vi "SRXConfigLimitSwitchSingle.vi"(0 "PhoenixMotorControlDevRefIn":T1={"DeviceStatus"={"status"=FALSE, "code"=0, "source"=""}, "Type"=enum."PWM", "PWM"={"PWM Channel"=enum."PWM 1", "DeadBand"={"Name"="", "maxPositivePwm"=0, "minPositivePwm"=0, "centerPwm"=0, "maxNegativePwm"=0, "minNegativePwm"=0, "angularRange"=0}}, "CAN"={"Device Number"=0, "SetOutput VI Ref"=variant(enum8{"Percent VBus", "Current", "Speed", "Position", "Voltage"} enum."Percent VBus"), "GetOutput VI Ref"=variant(refnum<k1> refnum), "Enable VI Ref"=variant(dbl 12.0), "Disable VI Ref"=variant(enum8{"Percent VBus", "Speed", "Position", "Slave", "Unchanged / Invalid", "Voltage Compensation", "Current", "Motion Profile"} enum."Percent VBus"), "Data"=variant}, "Invert"=FALSE, "DIO PWM"={"PWM \"Enable\" Channel"=enum."Invalid", "DIOChannel"=enum."Invalid", "PWM Rate"=0.0}}, 5 "MotorConfig":T6={"CAN Address"=0, "Invert"=FALSE, "InvertSensor"=FALSE, "Unit Conversion Factor"=0.0, "Brake Mode"=enum."Override to Brake", "Reverse Limt Switch Mode"=enum."Disabled", "Forward Limt Swith Mode"=enum."Disabled", "PWM Channel"=enum."Invalid", "Motor Controller Type"=enum."Talon SRX"}, 11 "error in (no error)":errorcluster) -> (4 "PhoenixMotorControlDevRefOut":T1={"DeviceStatus"={"status"=FALSE, "code"=0, "source"=""}, "Type"=enum."PWM", "PWM"={"PWM Channel"=enum."PWM 1", "DeadBand"={"Name"="", "maxPositivePwm"=0, "minPositivePwm"=0, "centerPwm"=0, "maxNegativePwm"=0, "minNegativePwm"=0, "angularRange"=0}}, "CAN"={"Device Number"=0, "SetOutput VI Ref"=variant(enum8{"Percent VBus", "Current", "Speed", "Position", "Voltage"} enum."Percent VBus"), "GetOutput VI Ref"=variant(refnum<k1> refnum), "Enable VI Ref"=variant(dbl 12.0), "Disable VI Ref"=variant(enum8{"Percent VBus", "Speed", "Position", "Slave", "Unchanged / Invalid", "Voltage Compensation", "Current", "Motion Profile"} enum."Percent VBus"), "Data"=variant}, "Invert"=FALSE, "DIO PWM"={"PWM \"Enable\" Channel"=enum."Invalid", "DIOChannel"=enum."Invalid", "PWM Rate"=0.0}}, 15 "error out":errorcluster)   [LabVIEW 2017]
uses:
  TypeDefs/ConfigComponents/Config_Motor.ctl
  <vilib>/Rock Robotics/WPI/ThirdParty/Phoenix-LabVIEW/Motor Controller/Controls/CTRE_Phoenix_MotorControl_NeutralMode.ctl
  <vilib>/Rock Robotics/WPI/ThirdParty/Phoenix-LabVIEW/Motor Controller/Controls/CTRE_Phoenix_MotorControl_LimitSwitchNormal.ctl
  <vilib>/Rock Robotics/SystemInterfaces/DIO/FPGA_DIOPWMChannel.ctl
  TypeDefs/ConfigComponents/Config_MotorCtrlType.ctl
  <vilib>/Rock Robotics/WPI/MotorControl/WPI_MotorControlDeviceRef.ctl
  <vilib>/Rock Robotics/WPI/MotorControl/WPI_MotorControlType.ctl
  <vilib>/Rock Robotics/WPI/PWM/WPI_PWMDeadband.ctl
  <vilib>/Rock Robotics/SystemInterfaces/DIO/FPGA_DIOChannel.ctl
  <vilib>/Rock Robotics/WPI/ThirdParty/Phoenix-LabVIEW/Motor Controller/Controls/CTRE_Phoenix_MotorControl_LimitSwitchSource_Local.ctl
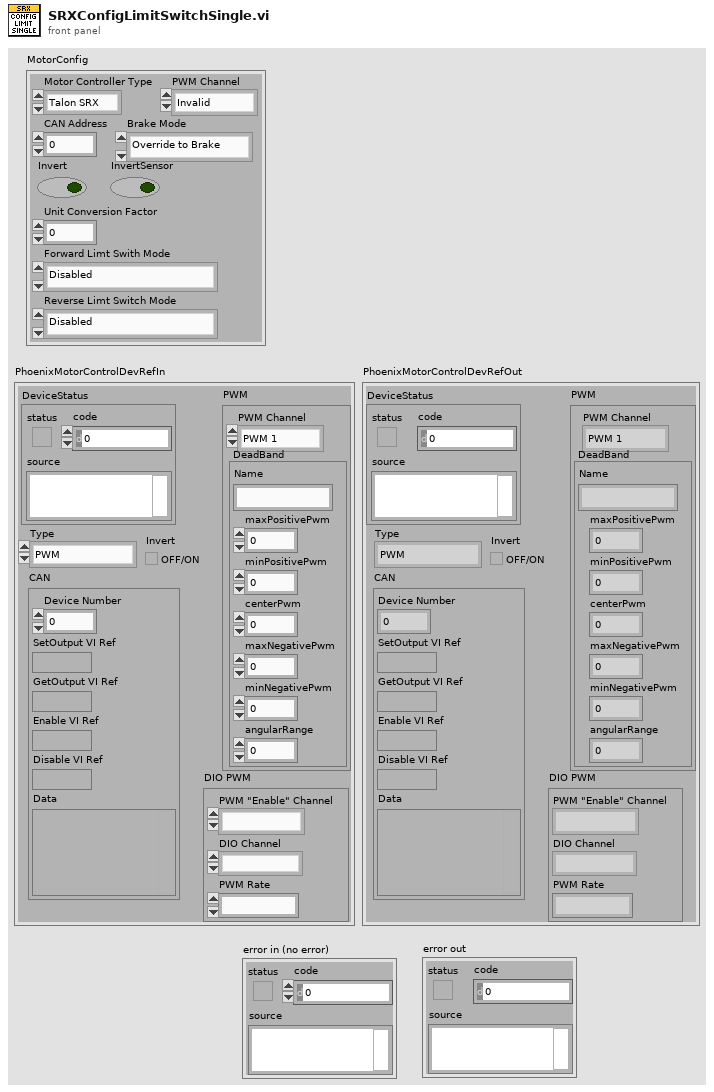
[diagram p1: front panel]
types:
  T1 = typedef "WPI_MotorControlDeviceRef.ctl" = cluster{"DeviceStatus":errorcluster, "Type":T2, "PWM":cluster{"PWM Channel":T3, "DeadBand":T4}, "CAN":cluster{"Device Number":u8, "SetOutput VI Ref":variant, "GetOutput VI Ref":variant, "Enable VI Ref":variant, "Disable VI Ref":variant, "Data":variant}, "Invert":bool, "DIO PWM":cluster{"PWM \"Enable\" Channel":T3, "DIOChannel":T5, "PWM Rate":dbl}}
  T2 = typedef "WPI_MotorControlType.ctl" = enum16{"PWM", "CAN", "DIO PWM"}
  T3 = typedef "FPGA_DIOPWMChannel.ctl" = enum8{"PWM 0", "PWM 1", "PWM 2", "PWM 3", "PWM 4", "PWM 5", "PWM 6", "PWM 7", "PWM 8", "PWM 9", "PWM MXP 0", "PWM MXP 1", "PWM MXP 2", "PWM MXP 3", "PWM MXP 4", "PWM MXP 5", "PWM MXP 6", "PWM MXP 7", "PWM MXP 8", "PWM MXP 9", "Invalid"}
  T4 = typedef "WPI_PWMDeadband.ctl" = cluster{"Name":string, "maxPositivePwm":i32, "minPositivePwm":i32, "centerPwm":i32, "maxNegativePwm":i32, "minNegativePwm":i32, "angularRange":u16}
  T5 = typedef "FPGA_DIOChannel.ctl" = enum8{"DIO 0", "DIO 1", "DIO 2", "DIO 3", "DIO 4", "DIO 5", "DIO 6", "DIO 7", "DIO 8", "DIO 9", "DIO MXP 0", "DIO MXP 1", "DIO MXP 2", "DIO MXP 3", "DIO MXP 4", "DIO MXP 5", "DIO MXP 6", "DIO MXP 7", "DIO MXP 8", "DIO MXP 9", "DIO MXP 10", "DIO MXP 11", "DIO MXP 12", "DIO MXP 13", "DIO MXP 14", "DIO MXP 15", "SPI Port CS1", "SPI Port CS2", "SPI Port CS3", "SPI Port MISO", "SPI Port MOSI", "Invalid"}
  T6 = typedef "Config_Motor.ctl" = cluster{"CAN Address":u8, "Invert":bool, "InvertSensor":bool, "Unit Conversion Factor":dbl, "Brake Mode":T7, "Reverse Limt Switch Mode":T8, "Forward Limt Swith Mode":T8, "PWM Channel":T3, "Motor Controller Type":T9}
  T7 = typedef "CTRE_Phoenix_MotorControl_NeutralMode.ctl" = enum8{"EEPROMSetting", "Override to Coast", "Override to Brake"}
  T8 = typedef "CTRE_Phoenix_MotorControl_LimitSwitchNormal.ctl" = enum16{"Normally Open", "Normally Closed", "Disabled"}
  T9 = typedef "Config_MotorCtrlType.ctl" = enum16{"Disabled", "Talon SRX", "Talon SR"}
  T10 = typedef "CTRE_Phoenix_MotorControl_LimitSwitchSource_Local.ctl" = enum16{"Feedback Connector", "Remote Talon SRX", "Remote CANifier", "Deactivated"}
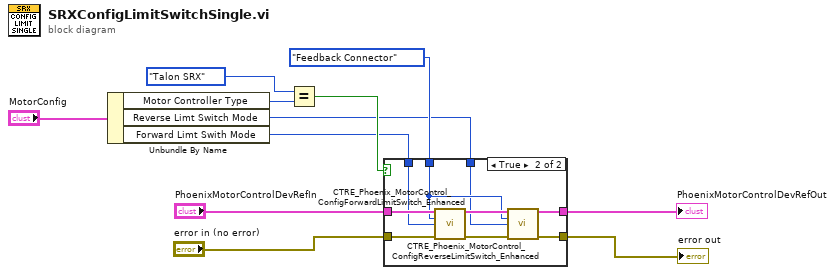
[diagram p0: block diagram]
diagram:
  n1 = Unbundle By Name("MotorConfig") -> ("Motor Controller Type"=w5:T9, "Reverse Limt Switch Mode"=w2:T8, "Forward Limt Swith Mode"=w1:T8)
  n2 = Equal?(x=Config_MotorCtrlType."Talon SRX", y=w5) -> (x = y?=w3:bool)
  n3 = case shown="True" w3 {
    tunnel: "PhoenixMotorControlDevRefIn" -> [w13 w20]
    tunnel: [w13 w19] -> w10
    tunnel: "error in (no error)" -> [w12 w18]
    tunnel: [w12 w17] -> w8
    tunnel: CTRE_Phoenix_MotorControl_LimitSwitchSource_Local."Feedback Connector" ("Limit Switch Source") -> [_ w16]
    tunnel: w2 -> [_ w15]
    tunnel: w1 -> [_ w14]
    frame False {
    }
    frame True {
      n4 = call <vilib>:"CTRE_Phoenix_MotorControl_ConfigForwardLimitSwitch_Enhanced.vi"("PhoenixMotorControlDevRef"=w20, "Limit Switch Source"=w16, "NormallyOpenOrClosed"=w14, "error in (no error)"=w18) -> ("PhoenixMotorControlDevRef"=w21:T1, "error out"=w22:errorcluster)  [unwired: 10 in]
      n5 = call <vilib>:"CTRE_Phoenix_MotorControl_ConfigReverseLimitSwitch_Enhanced.vi"("PhoenixMotorControlDevRef"=w21, "Limit Switch Source"=w16, "NormallyOpenOrClosed"=w15, "error in (no error)"=w22) -> ("PhoenixMotorControlDevRef"=w19:T1, "error out"=w17:errorcluster)  [unwired: 10 in]
    }
  }
  "PhoenixMotorControlDevRefOut" <- w10
  "error out" <- w8
